vi "Clusters.vi"(10 "Signal":T1) -> ()   [LabVIEW 2023]
panel:
  out "Sample Rate":dbl
  out "Device Name":string
  out "Samples":dbl[](array[numeric])
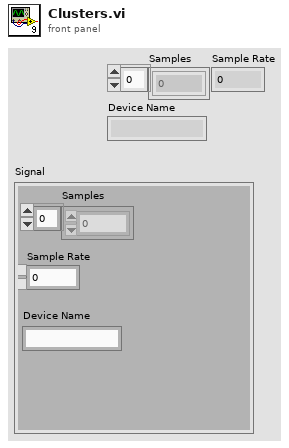
[diagram p1: front panel]
types:
  T1 = cluster{"Samples":dbl[], "Sample Rate":dbl, "Device Name":string}
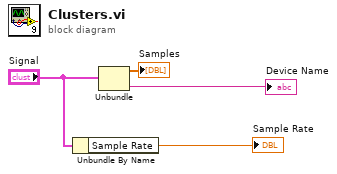
[diagram p0: block diagram]
diagram:
  n1 = Unbundle By Name("Signal") -> ("Sample Rate"=→"Sample Rate":dbl)
  n2 = Unbundle("Signal") -> ("Samples"=→"Samples":dbl[], "Device Name"=→"Device Name":string)  [unwired: 1 out]
